vi "aggiornamento.vi"() -> ()   [LabVIEW 2021]
panel:
  in  "fl2":bool
  in  "stop":bool
  in  "fl1":bool
  in  "start":bool
  out "ind":bool
  out "avn":bool
  out "led":bool
  in  "Enum":T1(ring)
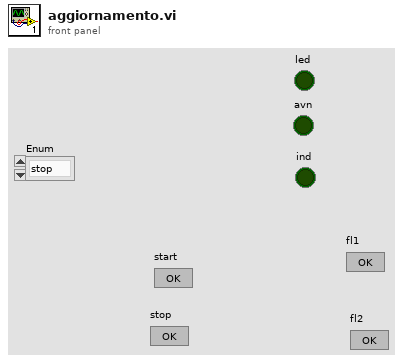
[diagram p1: front panel]
types:
  T1 = enum16{"stop", "attesa", "avanti", "indietro", "timer", "prelievo"}
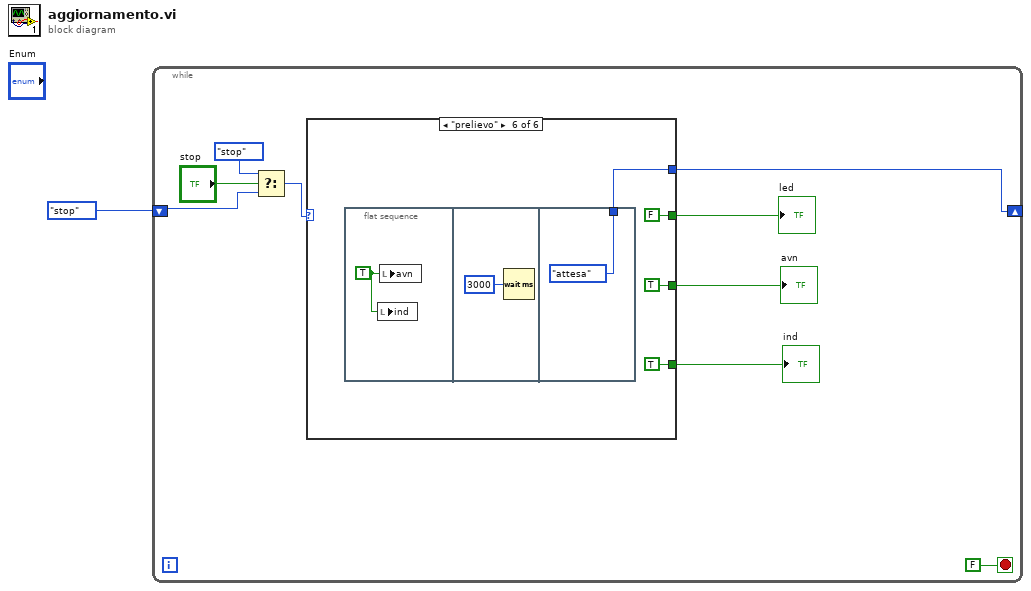
[diagram p0: block diagram]
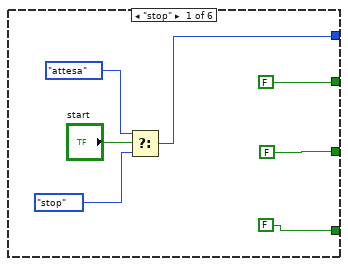
[diagram p2: hidden frame]
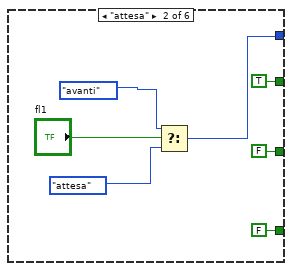
[diagram p3: hidden frame]
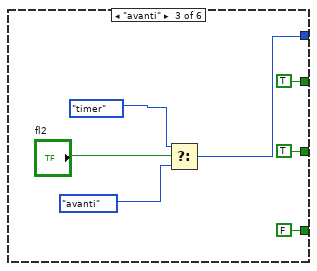
[diagram p4: hidden frame]
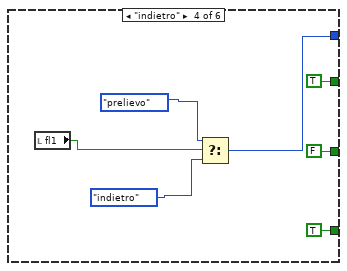
[diagram p5: hidden frame]
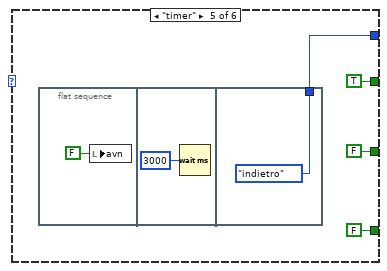
[diagram p6: hidden frame]
diagram:
  n1 = while {
    shift-right: [w7] -> _
    shift-left: T1."stop" ("Enum") -> [w3]
    stop <- FALSE stop-if-true
    n2 = Select(t=T1."stop" ("Enum"), s="stop", f=w3) -> (s? t:f=w2:T1)
    n3 = case shown="\"prelievo\"" w2 {
      tunnel: [FALSE TRUE TRUE TRUE TRUE FALSE] -> w10
      tunnel: [FALSE FALSE TRUE FALSE FALSE TRUE] -> w9
      tunnel: [FALSE FALSE FALSE TRUE FALSE TRUE] -> w8
      tunnel: [w13 w20 w25 w34 w39 w46] -> w7
      frame "stop" {
        n4 = Select(t=T1."attesa" ("Enum"), s="start", f=T1."stop" ("Enum")) -> (s? t:f=w13:T1)
      }
      frame "attesa" {
        n5 = Select(t=T1."avanti" ("Enum"), s="fl1", f=T1."attesa" ("Enum")) -> (s? t:f=w20:T1)
      }
      frame "avanti" {
        n6 = Select(t=T1."timer" ("Enum"), s="fl2", f=T1."avanti" ("Enum")) -> (s? t:f=w25:T1)
      }
      frame "indietro" {
        n7 = local read "fl1"() -> (w35:bool)
        n8 = Select(t=T1."prelievo" ("Enum"), s=w35, f=T1."indietro" ("Enum")) -> (s? t:f=w34:T1)
      }
      frame "timer" {
        n9 = flat-sequence {
          tunnel: [T1."indietro" ("Enum")] -> w39
          frame #0 {
            n10 = local write "avn"(FALSE ("avn")) -> ()
          }
          frame #1 {
            n11 = Wait (ms)(milliseconds to wait=u32 3000) -> ()  [unwired: 1 out]
          }
          frame #2 {
          }
        }
      }
      frame "prelievo" {
        n12 = flat-sequence {
          tunnel: [T1."attesa" ("Enum")] -> w46
          frame #0 {
            w50 = TRUE ("avn")
            n13 = local write "ind"(w50) -> ()
            n14 = local write "avn"(w50) -> ()
          }
          frame #1 {
            n15 = Wait (ms)(milliseconds to wait=u32 3000) -> ()  [unwired: 1 out]
          }
          frame #2 {
          }
        }
      }
    }
    "avn" <- w9
    "ind" <- w8
    "led" <- w10
  }
